vi "CF-calibration_filepath.vi"(11 "Input path":string) -> (2 "Common Path + input":path, 3 "calibration Path":path)   [LabVIEW 2020, in "CF-common_features.lvlib"]
uses:
  CF-common_features.lvlib
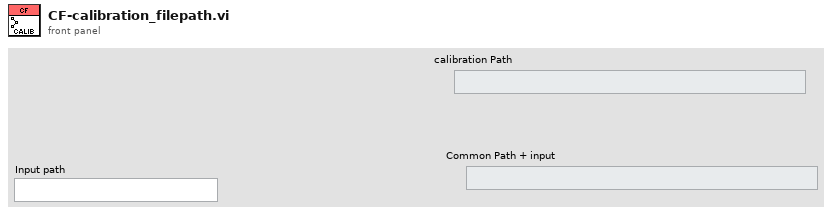
[diagram p1: front panel]
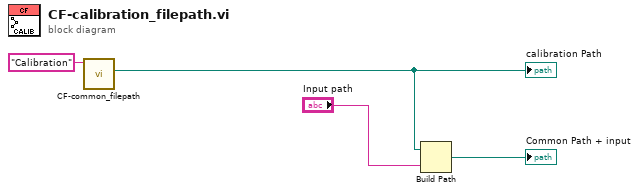
[diagram p0: block diagram]
diagram:
  n1 = call "CF-common_filepath.vi"("Input path"="Calibration") -> ("Common Path + input"=w2:path)  [unwired: 9 in, 1 out]
  "calibration Path" <- w2
  n2 = Build Path(base path=w2, name or relative path="Input path") -> (appended path=→"Common Path + input":path)
